vi "LINC Register Common Commands.vi"(8 "error in":errorcluster, 11 "LINC session":refnum<class "LINC.lvclass">) -> (0 "error out":errorcluster, 3 "dup LINC session":refnum<class "LINC.lvclass">)   [LabVIEW 2018, in "STEPkgDriver_LINC.lvlib" / "LINC.lvclass"]
uses:
  LINC.lvclass
panel:
  in  "common commands":T1
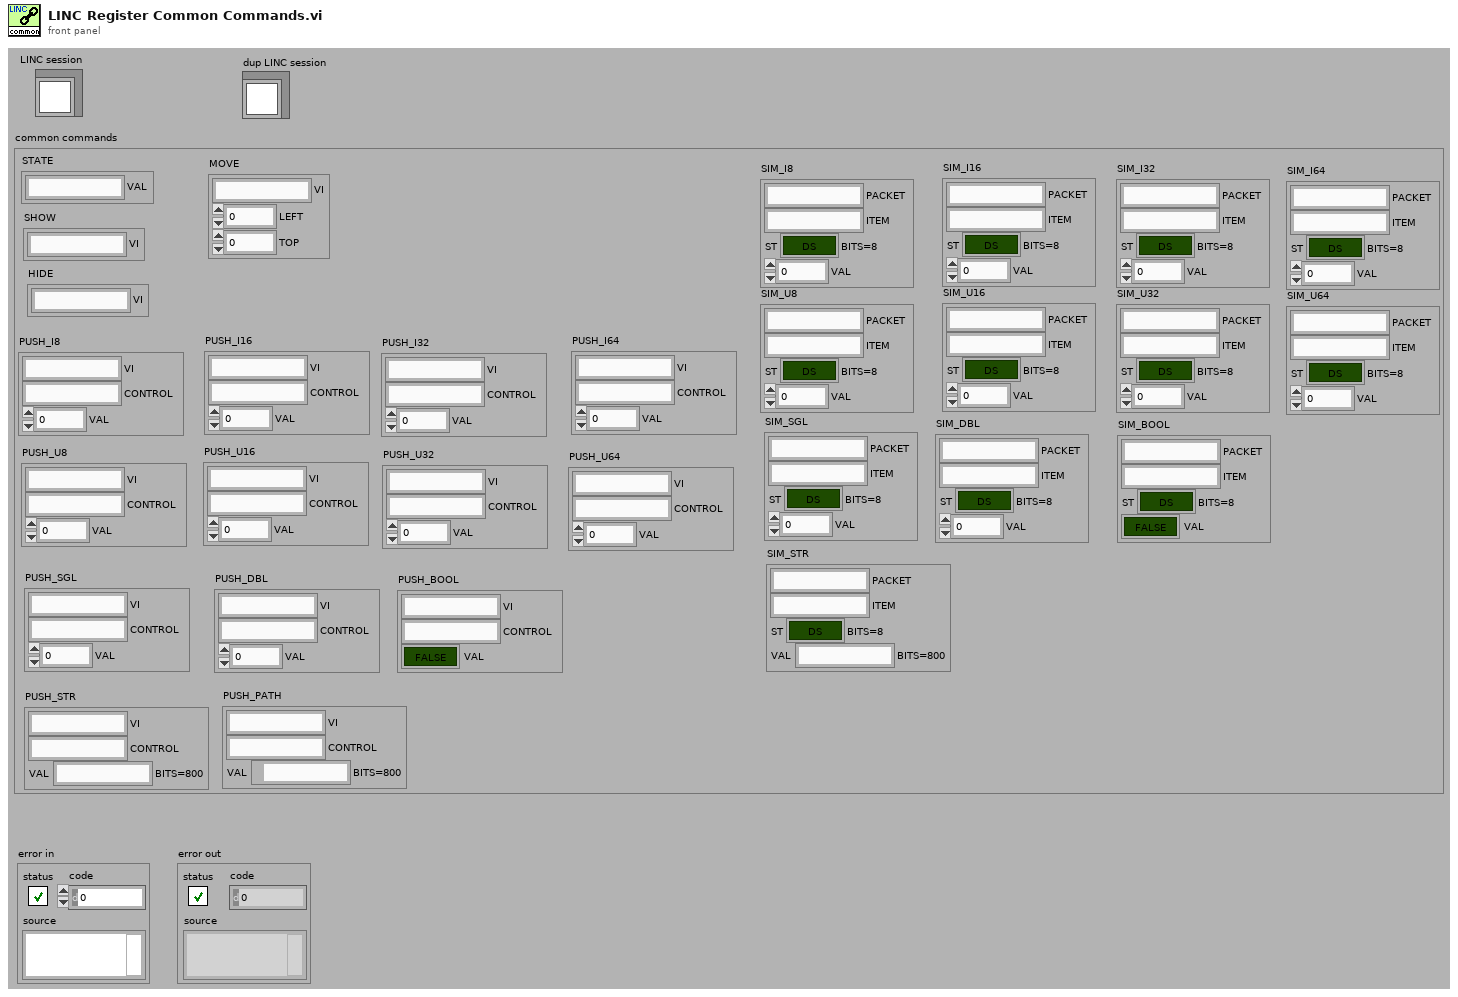
[diagram p1: front panel]
types:
  T1 = cluster{"PUSH_I8":cluster{"VI":string, "CONTROL":string, "VAL":i8}, "PUSH_I16":cluster{"VI":string, "CONTROL":string, "VAL":i16}, "PUSH_I32":cluster{"VI":string, "CONTROL":string, "VAL":i32}, "PUSH_I64":cluster{"VI":string, "CONTROL":string, "VAL":i64}, "PUSH_U8":cluster{"VI":string, "CONTROL":string, "VAL":u8}, "PUSH_U16":cluster{"VI":string, "CONTROL":string, "VAL":u16}, "PUSH_U32":cluster{"VI":string, "CONTROL":string, "VAL":u32}, "PUSH_U64":cluster{"VI":string, "CONTROL":string, "VAL":u64}, "PUSH_SGL":cluster{"VI":string, "CONTROL":string, "VAL":sgl}, "PUSH_DBL":cluster{"VI":string, "CONTROL":string, "VAL":dbl}, "PUSH_BOOL":cluster{"VI":string, "CONTROL":string, "VAL":bool}, "PUSH_STR":cluster{"VI":string, "CONTROL":string, "VAL":string}, "PUSH_PATH":cluster{"VI":string, "CONTROL":string, "VAL":path}, "STATE":cluster{"VAL":string}, "SHOW":cluster{"VI":string}, "HIDE":cluster{"VI":string}, "MOVE":cluster{"VI":string, "LEFT":i16, "TOP":i16}, "SIM_I8":cluster{"PACKET":string, "ITEM":string, "ST":bool, "VAL":i8}, "SIM_I16":cluster{"PACKET":string, "ITEM":string, "ST":bool, "VAL":i16}, "SIM_I32":cluster{"PACKET":string, "ITEM":string, "ST":bool, "VAL":i32}, "SIM_I64":cluster{"PACKET":string, "ITEM":string, "ST":bool, "VAL":i64}, "SIM_U8":cluster{"PACKET":string, "ITEM":string, "ST":bool, "VAL":u8}, "SIM_U16":cluster{"PACKET":string, "ITEM":string, "ST":bool, "VAL":u16}, "SIM_U32":cluster{"PACKET":string, "ITEM":string, "ST":bool, "VAL":u32}, "SIM_U64":cluster{"PACKET":string, "ITEM":string, "ST":bool, "VAL":u64}, "SIM_SGL":cluster{"PACKET":string, "ITEM":string, "ST":bool, "VAL":sgl}, "SIM_DBL":cluster{"PACKET":string, "ITEM":string, "ST":bool, "VAL":dbl}, "SIM_BOOL":cluster{"PACKET":string, "ITEM":string, "ST":bool, "VAL":bool}, "SIM_STR":cluster{"PACKET":string, "ITEM":string, "ST":bool, "VAL":string}}
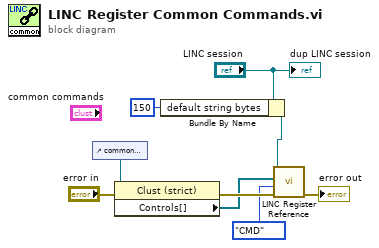
[diagram p0: block diagram]
diagram:
  n1 = control-ref of="common commands"() -> (w8:refnum<vi>)
  n2 = property class="Clust (strict)"(reference=w8, error in="error in") -> (error out=w7:errorcluster, "Controls[]"=w6:refnum<vi>[])  [unwired: 1 out]
  n3 = Bundle By Name(cluster="LINC session", "default string bytes"=150) -> (w2:refnum<class "LINC.lvclass">)
  n4 = call "LINC Register Reference.vi"("error in (no error)"=w7, "type (CMD)"=enum16{"CMD", "TLM", "CMD_HDR", "TLM_HDR"}."CMD", "controls"=w6, "LINC session"=w2) -> ("error out"=→"error out":errorcluster)  [unwired: 6 in, 1 out]
  "dup LINC session" <- "LINC session"
